vi "Export.vi"(8 "error in (no error)":errorcluster, 11 "Test Report in":refnum<class "Test Report.JUnit.lvclass">) -> (0 "error out":errorcluster, 3 "Test Report out":refnum<class "Test Report.JUnit.lvclass">)   [LabVIEW 2013, in "Caraya.lvlib" / "Test Report.JUnit.lvclass"]
uses:
  Test Report.JUnit.lvclass
  MsgSerializer.XML/MsgSerializer.XML.lvclass
  MsgSerializer.XML/format -- enum.ctl
  MsgSerializer.XML/MsgSerializer.XML.lvclass/MsgSerializer.XML.ctl
  Test Report.JUnit.lvclass/Test Report.JUnit.ctl
  Test Report/Test Report.lvclass/Test Report.ctl
  MsgSerializer/MsgSerializer.lvclass/MsgSerializer.ctl
  MsgSerializer.XML/Read Locale.vi
  MsgSerializer.XML/escapeXML.vi
  Test Report/Read MsgSerializer.vi
  Test Report/Test Report.lvclass
  Test Result/Test Result.lvclass
  Caraya.lvlib
panel:
  out "Serialized Message":string
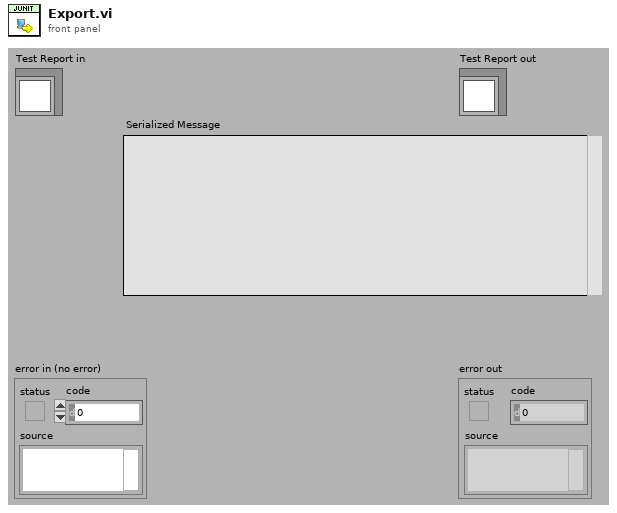
[diagram p1: front panel]
types:
  T1 = typedef "Caraya.lvlib/MsgSerializer.XML.lvclass/format -- enum.ctl" = enum16{"value", "tag", "property"}
  T2 = enum16{"open", "replace", "create", "open or create", "replace or create", "replace or create with confirmation"}
  T3 = cluster{"framework-name":string, "framework-version":string}
  T4 = typedef "Caraya.lvlib/Test Result.lvclass/Node Results (Extended).ctl" = cluster{"Test Node":T5, "Assertions":T7[]}
  T5 = typedef "Caraya.lvlib/Test Result.lvclass/Test Node (Extended).ctl" = cluster{"Test Registration":T6, "Defined":bool, "Passed":bool, "properties":variant}
  T6 = typedef "Caraya.lvlib/Test Result.lvclass/Test Registration Data.ctl" = cluster{"Name":string, "Call Chain":string[], "Time Stamp":timestamp, "Test ID":string, "Caller ID":string}
  T7 = typedef "Caraya.lvlib/Test Result.lvclass/Assert Event Data (Extended).ctl" = cluster{"name":string, "passed":bool, "call-chain":string[], "test-error":errorcluster, "timestamp":timestamp, "assert-id":string, "test-id":string, "time":dbl, "message":string, "properties":variant, "measurements":variant, "user-defined":variant}
  T8 = cluster{"Version String":string, "Name":string, "Copyright":string, "License":string}
  T9 = typedef "Caraya.lvlib/Test Report.JUnit.lvclass/testsuite -- cluster.ctl" = cluster{"name":string, "errors":u32, "skipped":u32, "tests":u32, "failures":u32, "time":dbl, "timestamp":timestamp, "call-chain":string[], "properties":variant}
  T10 = typedef "Caraya.lvlib/Test Report.JUnit.lvclass/extended -- cluster.ctl" = cluster{"classname":string, "name":string, "time":dbl, "skipped":bool, "failure":bool, "failure message":string, "failure description":string, "properties":variant, "measurements":variant, "user-defined":variant}
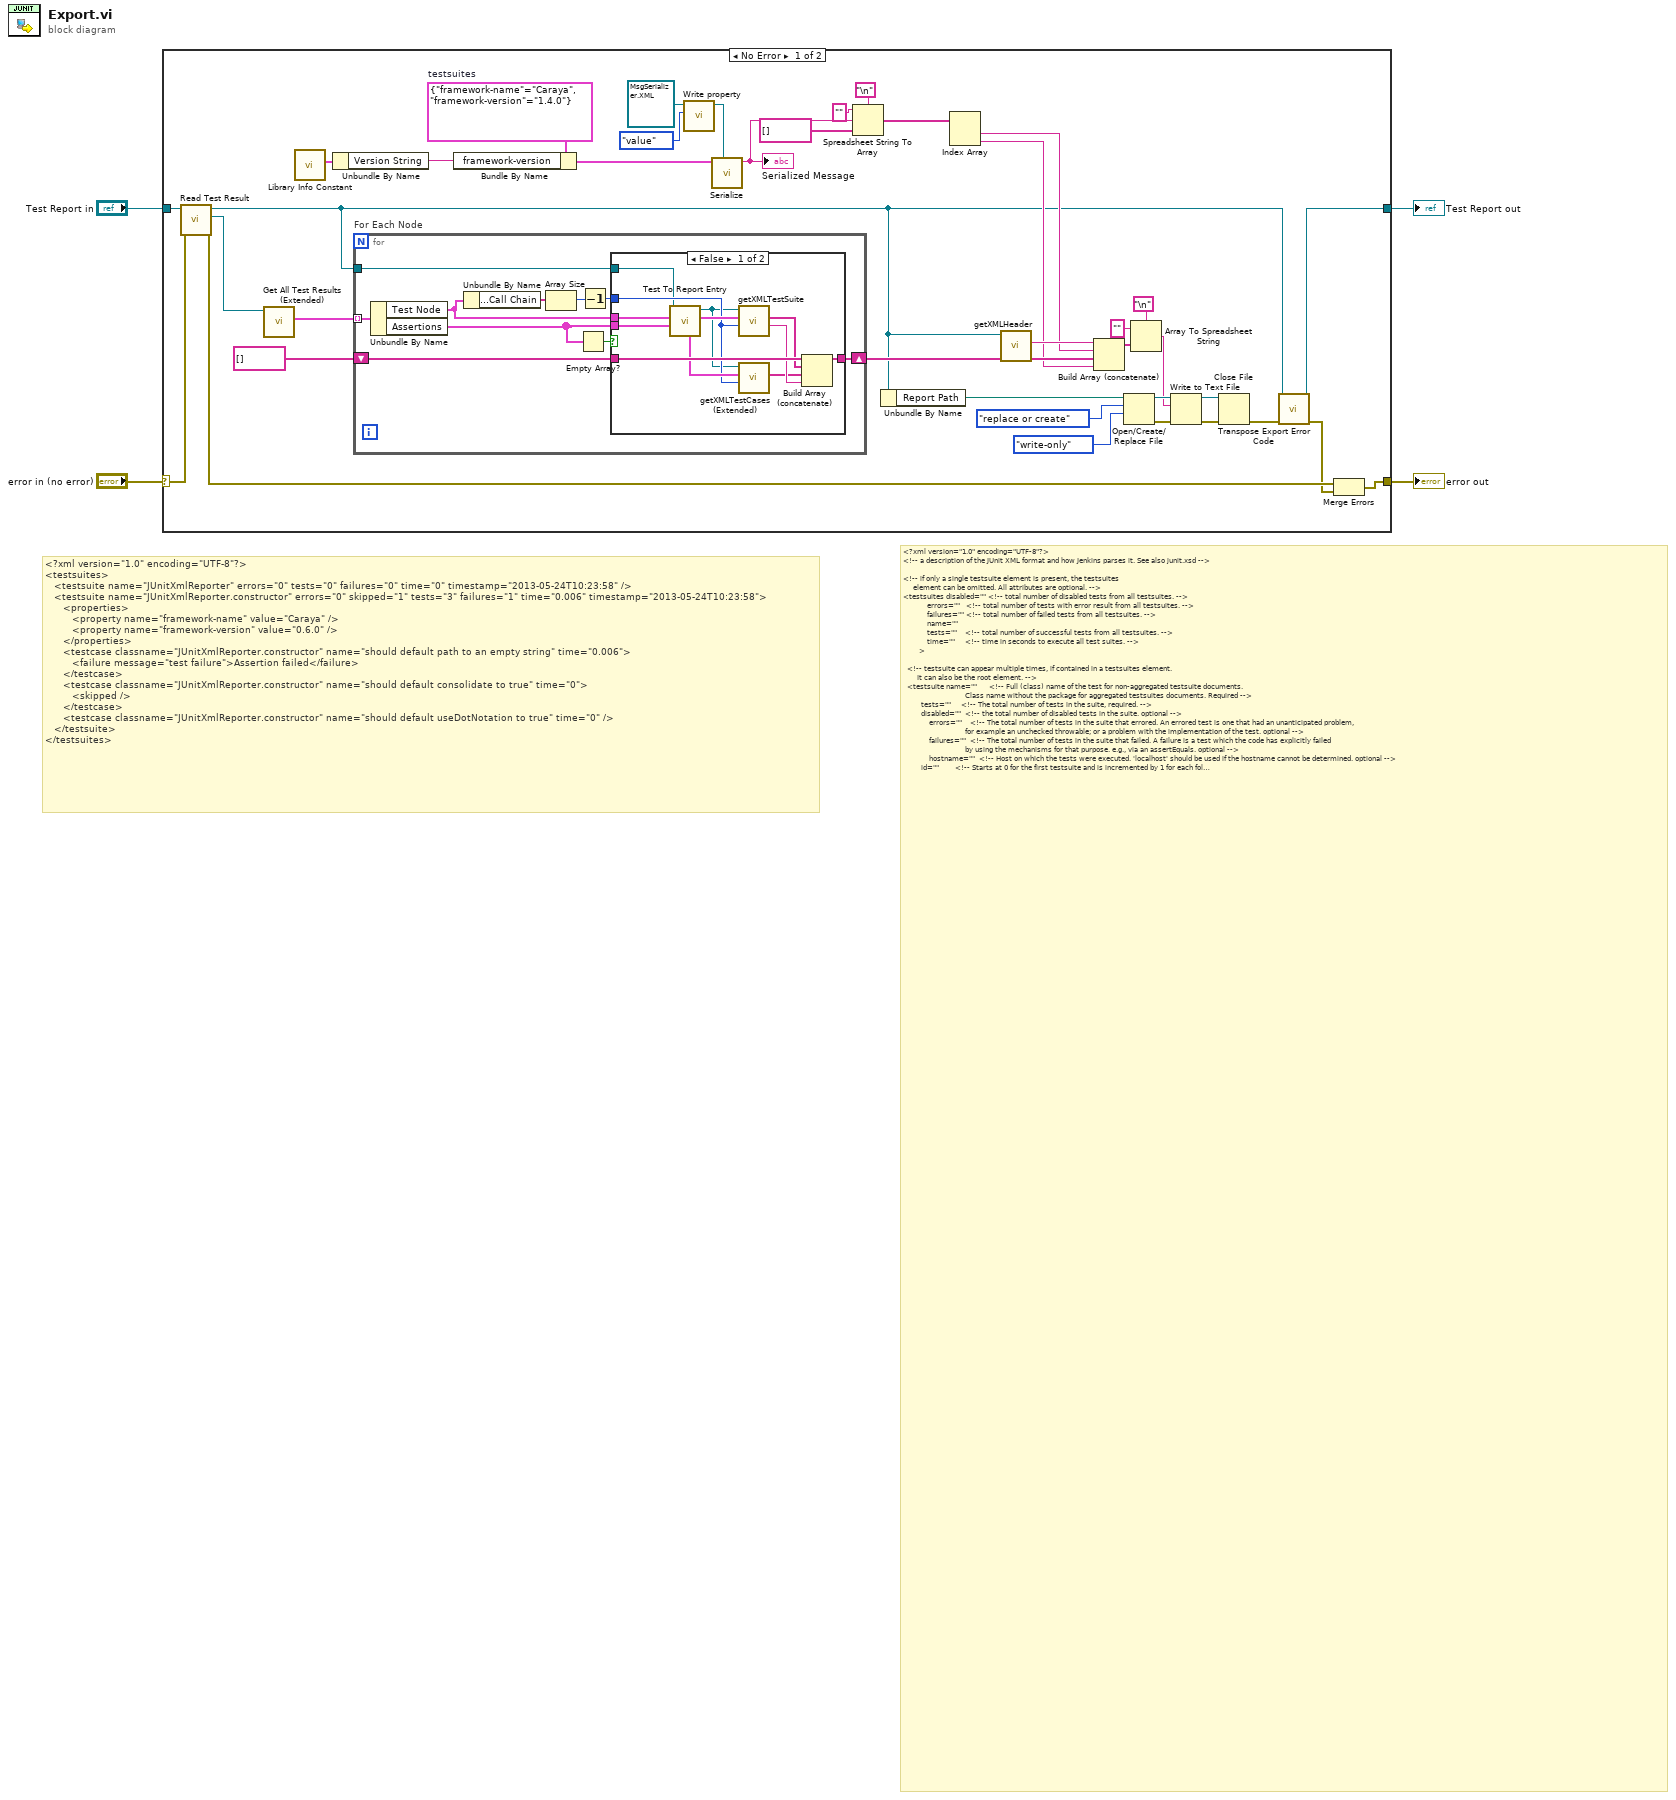
[diagram p0: block diagram]
diagram:
  # "<?xml version=\"1.0\" encoding=\"UTF-8\"?>\n<!-- a description of the JUnit XML format and how Jenkins parses it. See also junit.xsd -->\n\n<!-- if only a single testsuite element is present, the testsuites\n     element can be omitted. All attributes are optional. -->\n<testsuites disabled=\"\" <!-- total number of disabled tests from all testsuites. -->\n            errors=\"\"   <!-- total number of tests with error result from all testsuites. -->\n            failures=\"\" <!-- total number of failed tests from all testsuites. -->\n            name=\"\"\n            tests=\"\"    <!-- total number of successful tests from all testsuites. -->\n            time=\"\"     <!-- time in seconds to execute all test suites. -->\n        >\n\n  <!-- testsuite can appear multiple times, if contained in a testsuites element.\n       It can also be the root element. -->\n  <testsuite name=\"\"      <!-- Full (class) name of the test for non-aggregated testsuite documents.\n                               Class name without the package for aggregated testsuites documents. Required -->\n         tests=\"\"     <!-- The total number of tests in the suite, required. -->\n         disabled=\"\"  <!-- the total number of disabled tests in the suite. optional -->\n             errors=\"\"    <!-- The total number of tests in the suite that errored. An errored test is one that had an unanticipated problem,\n                               for example an unchecked throwable; or a problem with the implementation of the test. optional -->\n             failures=\"\"  <!-- The total number of tests in the suite that failed. A failure is a test which the code has explicitly failed\n                               by using the mechanisms for that purpose. e.g., via an assertEquals. optional -->\n             hostname=\"\"  <!-- Host on which the tests were executed. 'localhost' should be used if the hostname cannot be determined. optional -->\n         id=\"\"        <!-- Starts at 0 for the first testsuite and is incremented by 1 for each following testsuite -->\n         package=\"\"   <!-- Derived from testsuite/@name in the non-aggregated documents. optional -->\n         skipped=\"\"   <!-- The total number of skipped tests. optional -->\n         time=\"\"      <!-- Time taken (in seconds) to execute the tests in the suite. optional -->\n         timestamp=\"\" <!-- when the test was executed in ISO 8601 format (2014-01-21T16:17:18). Timezone may not be specified. optional -->\n         >\n\n    <!-- Properties (e.g., environment settings) set during test\n     execution. The properties element can appear 0 or once. -->\n    <properties>\n      <!-- property can appear multiple times. The name and value attributres are required. -->\n      <property name=\"\" value=\"\"/>\n    </properties>\n\n    <!-- testcase can appear multiple times, see /testsuites/testsuite@tests -->\n    <testcase name=\"\"       <!-- Name of the test method, required. -->\n          assertions=\"\" <!-- number of assertions in the test case. optional -->\n          classname=\"\"  <!-- Full class name for the class the test method is in. required -->\n          status=\"\"\n          time=\"\"       <!-- Time taken (in seconds) to execute the test. optional -->\n          >\n\n      <!-- If the test was not executed or failed, you can specify one\n           the skipped, error or failure elements. -->\n\n      <!-- skipped can appear 0 or once. optional -->\n      <skipped/>\n\n      <!-- Indicates that the test errored. An errored test is one\n           that had an unanticipated problem. For example an unchecked\n           throwable or a problem with the implementation of the\n           test. Contains as a text node relevant data for the error,\n           for example a stack trace. optional -->\n      <error message=\"\" <!-- The error message. e.g., if a java exception is thrown, the return value of getMessage() -->\n         type=\"\"    <!-- The type of error that occured. e.g., if a java execption is thrown the full class name of the exception. -->\n         ></error>\n\n      <!-- Indicates that the test failed. A failure is a test which\n       the code has explicitly failed by using the mechanisms for\n       that purpose. For example via an assertEquals. Contains as\n       a text node relevant data for the failure, e.g., a stack\n       trace. optional -->\n      <failure message=\"\" <!-- The message specified in the assert. -->\n           type=\"\"    <!-- The type of the assert. -->\n           ></failure>\n\n      <!-- Data that was written to standard out while the test was executed. optional -->\n      <system-out></system-out>\n\n      <!-- Data that was written to standard error while the test was executed. optional -->\n      <system-err></system-err>\n    </testcase>\n\n    <!-- Data that was written to standard out while the test suite was executed. optional -->\n    <system-out></system-out>\n    <!-- Data that was written to standard error while the test suite was executed. optional -->\n    <system-err></system-err>\n  </testsuite>\n</testsuites>"
  # "<?xml version=\"1.0\" encoding=\"UTF-8\"?>\n<testsuites>\n   <testsuite name=\"JUnitXmlReporter\" errors=\"0\" tests=\"0\" failures=\"0\" time=\"0\" timestamp=\"2013-05-24T10:23:58\" />\n   <testsuite name=\"JUnitXmlReporter.constructor\" errors=\"0\" skipped=\"1\" tests=\"3\" failures=\"1\" time=\"0.006\" timestamp=\"2013-05-24T10:23:58\">\n      <properties>\n         <property name=\"framework-name\" value=\"Caraya\" />\n         <property name=\"framework-version\" value=\"0.6.0\" />\n      </properties>\n      <testcase classname=\"JUnitXmlReporter.constructor\" name=\"should default path to an empty string\" time=\"0.006\">\n         <failure message=\"test failure\">Assertion failed</failure>\n      </testcase>\n      <testcase classname=\"JUnitXmlReporter.constructor\" name=\"should default consolidate to true\" time=\"0\">\n         <skipped />\n      </testcase>\n      <testcase classname=\"JUnitXmlReporter.constructor\" name=\"should default useDotNotation to true\" time=\"0\" />\n   </testsuite>\n</testsuites>"
  n1 = case shown="No Error" "error in (no error)" {
    selector: "error in (no error)" -> [w35 w67]
    tunnel: [w27 w67] -> w3
    tunnel: [w24 w66] -> w1
    tunnel: "Test Report in" -> [w23 w66]
    frame No Error {
      w15 = T3 {"framework-name"="Caraya", "framework-version"="1.4.0"}  # testsuites
      n2 = call "Read Test Result.vi"("error in (no error)"=w35, "Test Report in"=w23) -> ("error out"=w28:errorcluster, "Caraya.lvlib:Test Result.lvclass"=w22:refnum<class "Test Result.lvclass">, "Test Report out"=w5:refnum<class "Test Report.JUnit.lvclass">)  [unwired: 7 in]
      n3 = call "Get All Test Results (Extended).vi"("Test Result in"=w22) -> ("Test Results"=w21:T4[])  [unwired: 8 in, 2 out]
      n4 = call "Library Info Constant.vi"() -> ("Library Info Constant"=w14:T8)  [unwired: 11 in]
      n5 = Unbundle By Name(w14) -> ("Version String"=w16:string)
      n6 = for "For Each Node" {
        shift-right: [w47] -> w29
        shift-left: string[] [] ("appended array") -> [w52]
        tunnel: w21 -> [w51] mode=indexing
        tunnel: w5 -> [w45]
        n7 = Unbundle By Name(w51) -> ("Test Node"=w44:T5, "Assertions"=w43:T7[])
        n8 = Unbundle By Name(w44) -> ("Test Registration.Call Chain"=w48:string[])
        n9 = Array Size(array=w48) -> (size(s)=w50:i32)
        n10 = Empty Array?(array=w43) -> (empty?=w49:bool)
        n11 = Decrement(x=w50) -> (x-1=w46:i32)
        n12 = case shown="False" w49 {
          tunnel: w44 -> [w64 _]
          tunnel: w43 -> [w63 _]
          tunnel: w52 -> [w62 w65]
          tunnel: [w58 w65] -> w47
          tunnel: w46 -> [w56 _]
          tunnel: w45 -> [w54 _]
          frame False {
            n13 = call "Test To Report Entry.vi"("Asserts (aka. Test Cases)"=w63, "Node (aka. Test Suite)"=w64, "Test Report in"=w54) -> ("testsuite"=w61:T9, "Test Report"=w53:refnum<class "Test Report.JUnit.lvclass">, "testcases extended"=w57:T10[])  [unwired: 5 in, 1 out]
            n14 = call "getXMLTestSuite.vi"("indent level"=w56, "testsuite"=w61, "Test Report in"=w53) -> ("testsuite (end)"=w59:string, "testsuite (start)"=w60:string[])  [unwired: 6 in, 1 out]
            n15 = call "getXMLTestCases (Extended).vi"("indent level"=w56, "testcases"=w57, "Test Report in"=w53) -> ("XML Lines"=w55:string[])  [unwired: 7 in, 1 out]
            n16 = Build Array (concatenate)(w62, w60, w55, w59) -> (w58:string[])
          }
          frame True {
          }
        }
      }
      n17 = Bundle By Name(cluster=w15, "framework-version"=w16) -> (w17:T3)
      n18 = call "Write property.vi"("format"=format_--_enum."value", "MsgSerializer.XMLProperty in"=refnum<class "MsgSerializer.XML.lvclass"> refnum ("Caraya.lvlib:MsgSerializer.XMLProperty.lvclass")) -> ("MsgSerializer.XMLProperty out"=w19:refnum<class "MsgSerializer.XML.lvclass">)  [unwired: 9 in]
      n19 = call-dynamic "Serialize.vi"("MsgSerializer"=w19, "Value"=w17) -> ("Serialized Message"=w11:string)  [unwired: 8 in, 1 out]
      "Serialized Message" <- w11
      n20 = Spreadsheet String To Array(delimiter (Tab)="\n", format string="", spreadsheet string=w11, array type (2D Dbl)=string[] [] ("appended array")) -> (array=w9:string[])
      n21 = Unbundle By Name(w5) -> ("Report Path"=w36:path)
      n22 = Index Array(array=w9) -> (element #1=w8:string, element #2=w7:string)  [unwired: 2 in]
      n23 = call "getXMLHeader.vi"("Test Report in"=w5) -> ("xml header"=w33:string)  [unwired: 10 in]
      n24 = Build Array (concatenate)(w33, w8, w29, w7) -> (w32:string[])
      n25 = Open/Create/Replace File(file path (use dialog)=w36, operation (0:open)=T2."replace or create", access (0:read/write)=enum16{"read/write", "read-only", "write-only"}."write-only") -> (refnum out=w40:refnum<file>, error out=w39:errorcluster)  [unwired: 3 in, 1 out]
      n26 = Array To Spreadsheet String(delimiter (Tab)="\n", array=w32, 3:"" ("format string")) -> (spreadsheet string=w34:string)
      n27 = Write to Text File(file (use dialog)=w40, text=w34, error in=w39) -> (refnum out=w38:refnum<file>, error out=w37:errorcluster)  [unwired: 1 in, 1 out]
      n28 = Close File(refnum=w38, error in=w37) -> (error out=w26:errorcluster)  [unwired: 1 out]
      n29 = call-dynamic "Transpose Export Error Code.vi"("error in (no error)"=w26, "Test Report"=w5) -> ("error out"=w25:errorcluster, "Test Report out"=w24:refnum<class "Test Report.JUnit.lvclass">)  [unwired: 8 in]
      n30 = Merge Errors(w28, w25) -> (w27:errorcluster)
    }
    frame Error {
    }
  }
  "error out" <- w3
  "Test Report out" <- w1
